vi "Write Processed PA Block.vi"(8 "error in (no error)":errorcluster, 10 "Processed PA Block":T1, 11 "RDS State in":refnum<class "RDS State.lvclass">) -> (0 "error out":errorcluster, 3 "RDS State out":refnum<class "RDS State.lvclass">)   [LabVIEW 2015]
uses:
  RDS State.lvclass
  Processed PA Block.ctl
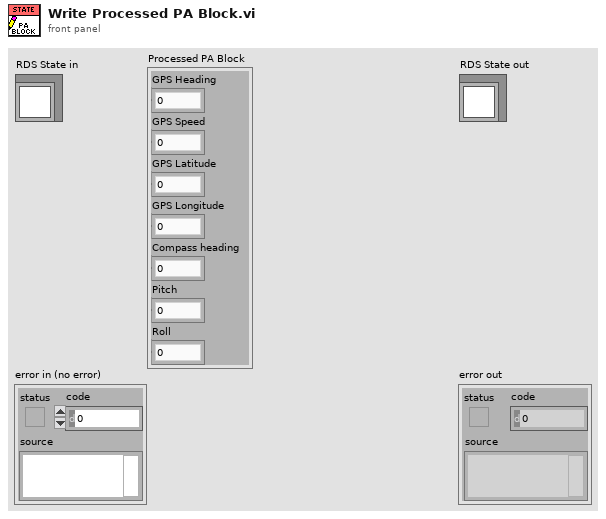
[diagram p1: front panel]
types:
  T1 = typedef "Processed PA Block.ctl" = cluster{"GPS Heading":dbl, "GPS Speed":dbl, "GPS Latitude":ext, "GPS Longitude":ext, "Compass heading":dbl, "Pitch":dbl, "Roll":dbl}
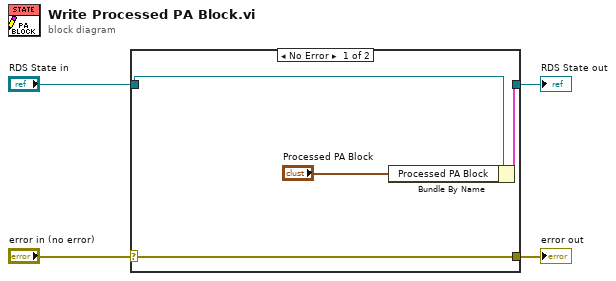
[diagram p0: block diagram]
diagram:
  n1 = case shown="No Error" "error in (no error)" {
    selector: "error in (no error)" -> [w8 w9]
    tunnel: [w8 w9] -> w3
    tunnel: [w6 w10] -> w1
    tunnel: "RDS State in" -> [w7 w10]
    frame No Error {
      n2 = Bundle By Name(cluster=w7, "Processed PA Block"="Processed PA Block") -> (w6:cluster{})
    }
    frame Error {
    }
  }
  "error out" <- w3
  "RDS State out" <- w1
